vi "Get device in.vi"(8 "error in (no error)":errorcluster caption="entrée d'erreur (pas d'erreur)", 11 "Class DIO NI en entrée":refnum<class "Class DIO NI.lvclass">) -> (0 "error out":errorcluster caption="sortie d'erreur", 2 "device in":tag caption="Address_Device", 3 "Class DIO NI en sortie":refnum<class "Class DIO NI.lvclass">)   [LabVIEW 2020, in "Library Instrument & Equipement.lvlib" / "Library DIO.lvlib" / "Class DIO NI.lvclass"]
uses:
  Class DIO NI.lvclass
  Class DIO NI.lvclass/Class DIO NI.ctl
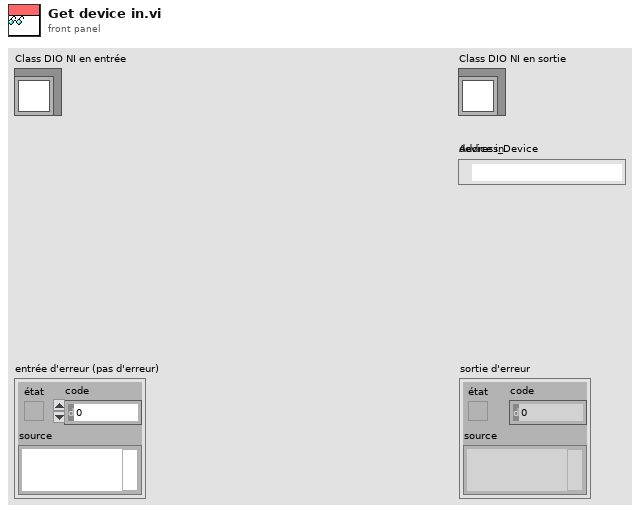
[diagram p1: front panel]
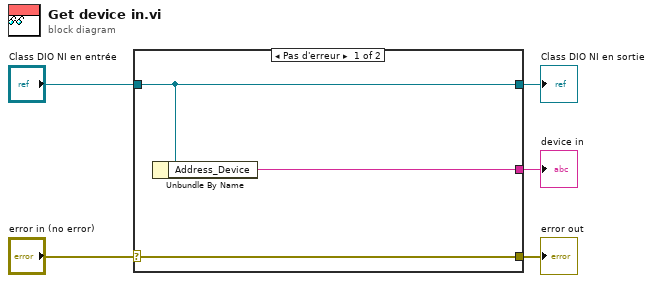
[diagram p0: block diagram]
diagram:
  n1 = case shown="Pas d'erreur" "error in (no error)" {
    selector: "error in (no error)" -> [w8 w9]
    tunnel: [w8 w9] -> w4
    tunnel: [w7 w10] -> w2
    tunnel: "Class DIO NI en entrée" -> [w7 w10]
    tunnel: [w6 _] -> w1
    frame No Error {
      n2 = Unbundle By Name(w7) -> ("Address_Device"=w6:tag)
    }
    frame Error {
    }
  }
  "error out" <- w4
  "Class DIO NI en sortie" <- w2
  "device in" <- w1
